vi "HamburgerMenu.SetPosition.vi"(7 "Caller VI Refnum":refnum<vi>, 8 "error in (no error)":errorcluster, 11 "Current VI Refnum":refnum<vi>) -> (0 "error out":errorcluster, 3 "Current VI Refnum out":refnum<vi>)   [LabVIEW 2019]
doc: "Copyright © 2006 James Kring, Inc. All rights reserved.\nMichael Aivaliotis michael.aivaliotis@jameskring.com\nalternate email: michael@aivaliotis.com\n\nThis library is provided \"AS IS\" , WITHOUT WARRANTIES OR \nCONDITIONS OF ANY KIND, either express or implied.\n\nJames Kring, Inc. -- http://www.jameskring.com"
panel:
  # "Copyright © 2014 JKI All rights reserved.\n\nFor more information contact: <info@jki.net>\n\nThis library is provided \"AS IS\" ,WITHOUT WARRANTIES OR \nCONDITIONS OF ANY KIND, either express or implied.\n\nJKI -- jki.net"
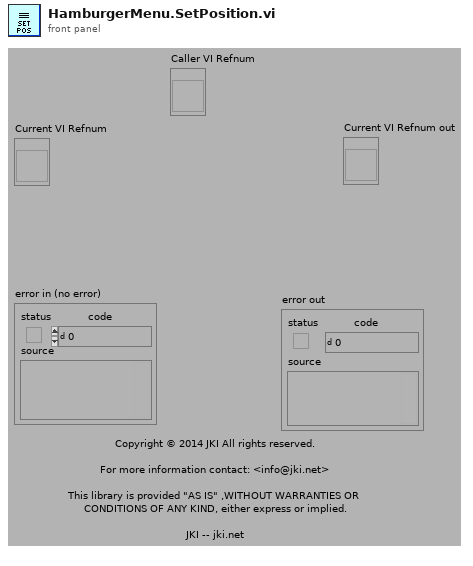
[diagram p1: front panel]
types:
  T1 = typedef "LVRectTypeDef.ctl" = cluster{"Left":i16, "Top":i16, "Right":i16, "Bottom":i16}
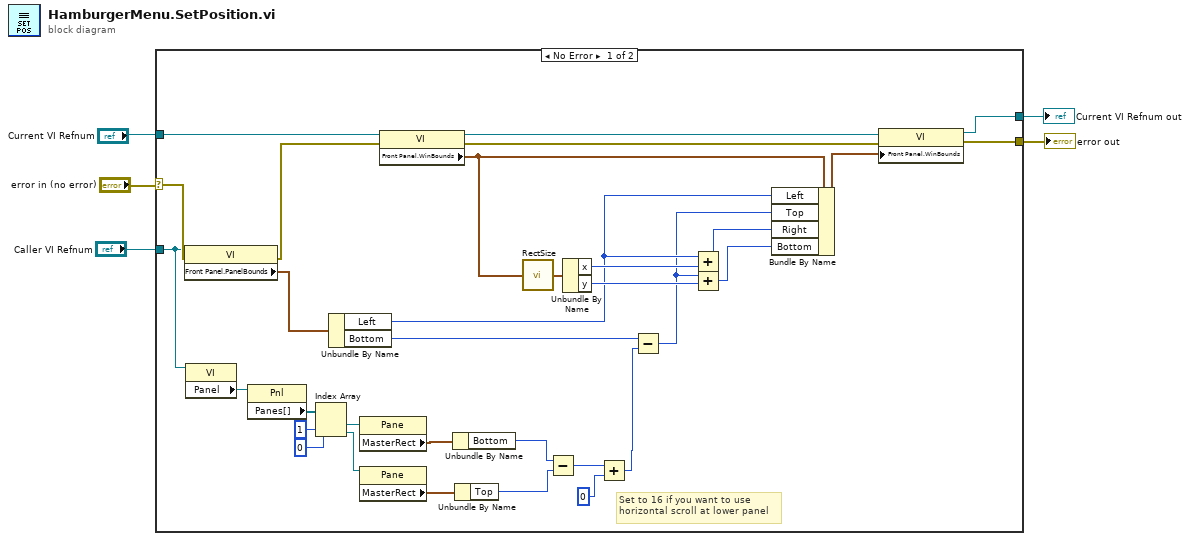
[diagram p0: block diagram]
diagram:
  n1 = case shown="No Error" "error in (no error)" {
    selector: "error in (no error)" -> [w25 w39]
    tunnel: [w36 w38] -> w5
    tunnel: "Current VI Refnum" -> [w35 w38]
    tunnel: [w31 w39] -> w3
    tunnel: "Caller VI Refnum" -> [w18 _]
    frame No Error {
      # "Set to 16 if you want to use\nhorizontal scroll at lower panel"
      n2 = property class="VI"(reference=w18, error in=w25) -> (error out=w24:errorcluster, "Front Panel.PanelBounds"=w23:T1)  [unwired: 1 out]
      n3 = property class="VI"(reference=w18) -> ("Panel"=w19:refnum<vi>)  [unwired: 1 in, 2 out]
      n4 = property class="Pnl"(reference=w19) -> ("Panes[]"=w20:refnum<vi>[])  [unwired: 1 in, 2 out]
      n5 = Index Array(array=w20, index #1=1 ("index"), index #2=0 ("index")) -> (element #1=w21:refnum<vi>, element #2=w14:refnum<vi>)
      n6 = Unbundle By Name(w23) -> ("Left"=w22:i16, "Bottom"=w16:i16)
      n7 = property class="Pane"(reference=w21) -> ("MasterRect"=w17:T1)  [unwired: 1 in, 2 out]
      n8 = property class="Pane"(reference=w14) -> ("MasterRect"=w13:T1)  [unwired: 1 in, 2 out]
      n9 = property class="VI"(reference=w35, error in=w24) -> (reference out=w33:refnum<vi>, error out=w37:errorcluster, "Front Panel.WinBounds"=w26:T1)
      n10 = Unbundle By Name(w17) -> ("Bottom"=w10:i16)
      n11 = Unbundle By Name(w13) -> ("Top"=w9:i16)
      n12 = call <vilib>:"RectSize.vi"("rect"=w26) -> ("point"=w32:cluster{"x":i16, "y":i16})
      n13 = Subtract(x=w10, y=w9) -> (x-y=w8:i16)
      n14 = Unbundle By Name(w32) -> ("x"=w30:i16, "y"=w28:i16)
      n15 = Add(x=w8, y=i16 0) -> (x+y=w7:i16)
      n16 = Subtract(x=w16, y=w7) -> (x-y=w15:i16)
      n17 = Add(x=w22, y=w30) -> (x+y=w29:i16)
      n18 = Add(x=w15, y=w28) -> (x+y=w27:i16)
      n19 = Bundle By Name(cluster=w26, "Left"=w22, "Top"=w15, "Right"=w29, "Bottom"=w27) -> (w34:T1)
      n20 = property class="VI"(reference=w33, error in=w37, "Front Panel.WinBounds"=w34) -> (reference out=w36:refnum<vi>, error out=w31:errorcluster)
    }
    frame Error {
    }
  }
  "error out" <- w3
  "Current VI Refnum out" <- w5
